vi "Ke2400 Initialize.vi"(7 "Serial Configuration":T1 {"Stop Bits" items=["1.0"=10, "1.5"=15, "2.0"=20]; "Data Bits" items=["7"=7, "8"=8]; "Parity" items=["None", "Odd", "Even", "Mark", "Space"]; "Flow Control" items=["None", "XON/XOFF", "RTS/CTX", "XON/XOFF & RTX/CTX", "DTR/DSR", "XON/XOFF & DTR/DSR"]; "Baud Rate" items=["300"=300, "600"=600, "1200"=1200, "2400"=2400, "4800"=4800, "9600"=9600, "19200"=19200]}, 8 "error in (no error)":errorcluster, 9 "Reset (True)":bool=TRUE, 10 "ID Query":bool=TRUE, 11 "VISA resource name":refnum<visa-resource-name>) -> (0 "error out":errorcluster, 3 "VISA resource name out":refnum<visa-resource-name>)   [LabVIEW 2012]
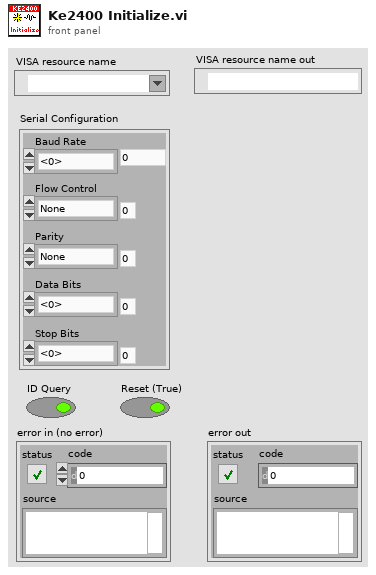
[diagram p1: front panel]
types:
  T1 = cluster{"Baud Rate":u32, "Flow Control":u16, "Parity":u16, "Data Bits":u16, "Stop Bits":u16}
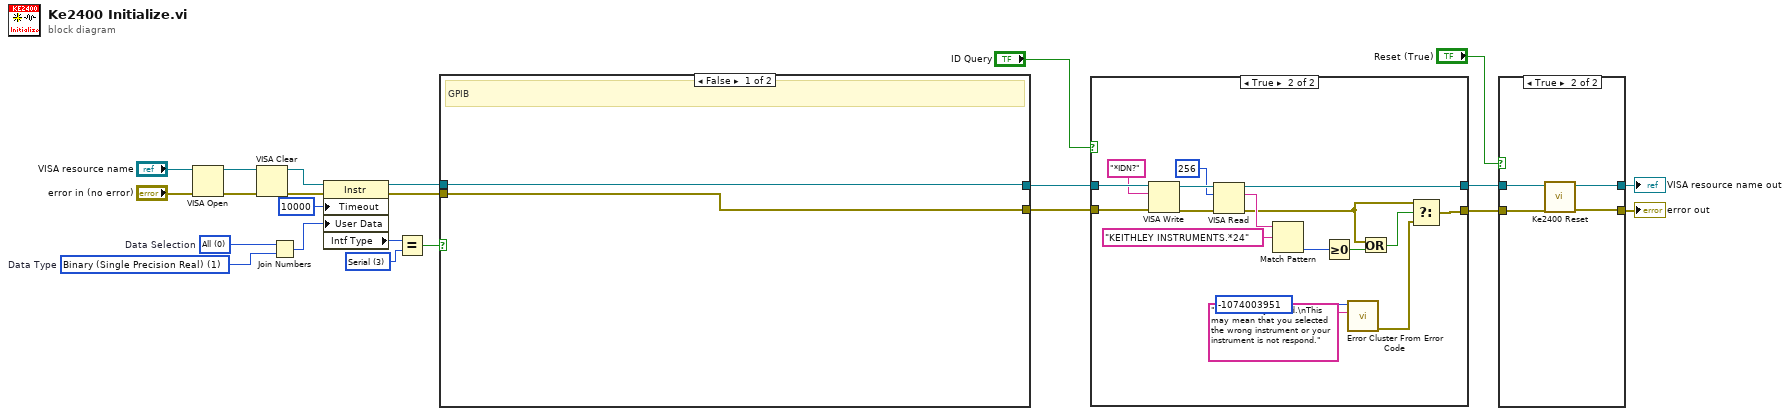
[diagram p0: block diagram]
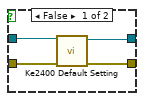
[diagram p2: hidden frame]
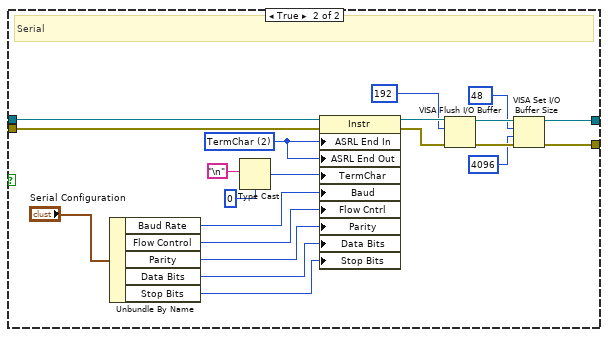
[diagram p4: hidden frame]
diagram:
  w10 = u16 3 items=["GPIB", "VXI", "GPIB-VXI", "Serial", "PXI", "TCPIP", "USB", "<Other>..."] ("Type Control")
  w12 = u16 1 items=["ASCII", "Binary (Single Precision Real)"]  # Data Type
  w13 = u16 0 items=["All", "Volt and Amp", "Volt", "Amp"]  # Data Selection
  n1 = VISA Open(error in (no error)="error in (no error)", VISA resource name="VISA resource name") -> (VISA resource name=w23:refnum<visa-resource-name>, error out=w22:errorcluster)  [unwired: 3 in]
  n2 = VISA Clear(VISA resource name=w23, error in (no error)=w22) -> (VISA resource name out=w18:refnum<visa-resource-name>, error out=w19:errorcluster)
  n3 = Join Numbers(hi=w13, lo=w12) -> ((hi.lo)=w14:u32)
  n4 = property class="Instr"(reference=w18, error in=w19, "Timeout"=u32 10000 ("General Settings:Timeout Value"), "User Data"=w14) -> (reference out=w17:refnum<visa-resource-name>, error out=w16:errorcluster, "Intf Type"=w11:u16)
  n5 = Equal?(x=w11, y=w10) -> (x = y?=w9:bool)
  n6 = case shown="False" w9 {
    tunnel: w17 -> [w25 w44]
    tunnel: w16 -> [w24 w45]
    tunnel: [w24 w27] -> w7
    tunnel: [w25 w26] -> w6
    frame False {
      # "GPIB"
    }
    frame True {
      w43 = u16 2 items=["None", "LastBit", "TermChar"] ("Set Serial End Mode for Read")
      # "Serial"
      n7 = Unbundle By Name("Serial Configuration") -> ("Baud Rate"=w39:u32, "Flow Control"=w38:u16, "Parity"=w37:u16, "Data Bits"=w36:u16, "Stop Bits"=w35:u16)
      n8 = Type Cast(type=u8 0, x="\n") -> (*(type *) &x=w40:u8)
      n9 = property class="Instr"(reference=w44, error in=w45, "ASRL End In"=w43, "ASRL End Out"=w43, "TermChar"=w40, "Baud"=w39, "Flow Cntrl"=w38, "Parity"=w37, "Data Bits"=w36, "Stop Bits"=w35) -> (reference out=w34:refnum<visa-resource-name>, error out=w33:errorcluster)
      n10 = VISA Flush I/O Buffer(VISA resource name=w34, mask (16)=u16 192 ("Numeric"), error in (no error)=w33) -> (VISA resource name out=w30:refnum<visa-resource-name>, error out=w31:errorcluster)
      n11 = VISA Set I/O Buffer Size(VISA resource name=w30, mask (16)=u16 48 ("Numeric"), size (4096)=u32 4096, error in (no error)=w31) -> (VISA resource name out=w26:refnum<visa-resource-name>, error out=w27:errorcluster)
    }
  }
  n12 = case shown="True" "ID Query" {
    tunnel: w7 -> [w48 w65]
    tunnel: w6 -> [w47 w64]
    tunnel: [w48 w50] -> w3
    tunnel: [w47 w49] -> w4
    frame False {
    }
    frame True {
      n13 = VISA Write(VISA resource name=w64, write buffer="*IDN?", error in (no error)=w65) -> (VISA resource name out=w61:refnum<visa-resource-name>, error out=w62:errorcluster)  [unwired: 1 out]
      n14 = VISA Read(VISA resource name=w61, byte count=u32 256, error in (no error)=w62) -> (VISA resource name out=w49:refnum<visa-resource-name>, read buffer=w59:string, error out=w55:errorcluster)  [unwired: 1 out]
      n15 = Match Pattern(string=w59, regular expression="KEITHLEY INSTRUMENTS.*24") -> (offset past match=w57:i32)  [unwired: 1 in, 3 out]
      n16 = Greater Or Equal To 0?(x=w57) -> (x >= 0?=w56:bool)
      n17 = call <vilib>:"Error Cluster From Error Code.vi"("error message (\"\")"="The ID Query Failed.\nThis may mean that you selected the wrong instrument or your instrument is not respond." ("error message (\"\")"), "error code (0)"=-1074003951 ("Numeric")) -> ("error out"=w51:errorcluster)  [unwired: 7 in]
      n18 = Or(x=w55, y=w56) -> (x .or. y?=w54:bool)
      n19 = Select(t=w55, s=w54, f=w51) -> (s? t:f=w50:errorcluster)
    }
  }
  n20 = case shown="True" "Reset (True)" {
    tunnel: w4 -> [w67 w73]
    tunnel: w3 -> [w69 w72]
    tunnel: [w68 w71] -> w2
    tunnel: [w66 w70] -> w1
    frame False {
      n21 = call "Ke2400 Default Setting.vi"("error in (no error)"=w69, "VISA resource name"=w67) -> ("error out"=w68:errorcluster, "VISA resource name out"=w66:refnum<visa-resource-name>)  [unwired: 8 in]
    }
    frame True {
      n22 = call "Ke2400 Reset.vi"("error in (no error)"=w72, "VISA resource name"=w73) -> ("error out"=w71:errorcluster, "VISA resource name out"=w70:refnum<visa-resource-name>)  [unwired: 8 in]
    }
  }
  "error out" <- w2
  "VISA resource name out" <- w1
